vi "ShootRole.vi"(7 "firstCall":bool=TRUE, 8 "error in (no error)":errorcluster, 9 "Robot":refnum<class "Robot.lvclass">, 10 "Game in":refnum<class "Game.lvclass">, 11 "ShootRole in":refnum<class "ShootRole.lvclass">) -> (0 "error out":errorcluster, 1 "Game out":refnum<class "Game.lvclass">, 2 "Robot out":refnum<class "Robot.lvclass">, 3 "ShootRole out":refnum<class "ShootRole.lvclass">)   [LabVIEW 2023, in "ShootRole.lvclass"]
uses:
  ShootRole.lvclass
  Game_class/Game.lvclass
  Robot_class/Robot.lvclass
  Role_class/Role.lvclass/Role.ctl
  ShootTactic_class/States.ctl
  Tacticbook_class/Tacticbook.lvclass/Tacticbook.ctl
  ShootTactic_class/ShootTactic.lvclass/ShootTactic.ctl
  Tacticbook_class/Read ShootTactic.vi
  ShootTactic_class/Read States.vi
  Tacticbook_class/Write ShootTactic.vi
  Role_class/Read Tacticbook.vi
  Role_class/Write Tacticbook.vi
  Role_class/Write tactic_index.vi
  Role_class/Read RobotRef.vi
  Tacticbook_class/Tacticbook.lvclass
  ShootTactic_class/ShootTactic.lvclass
  ShootRole.lvclass/ShootRole.ctl
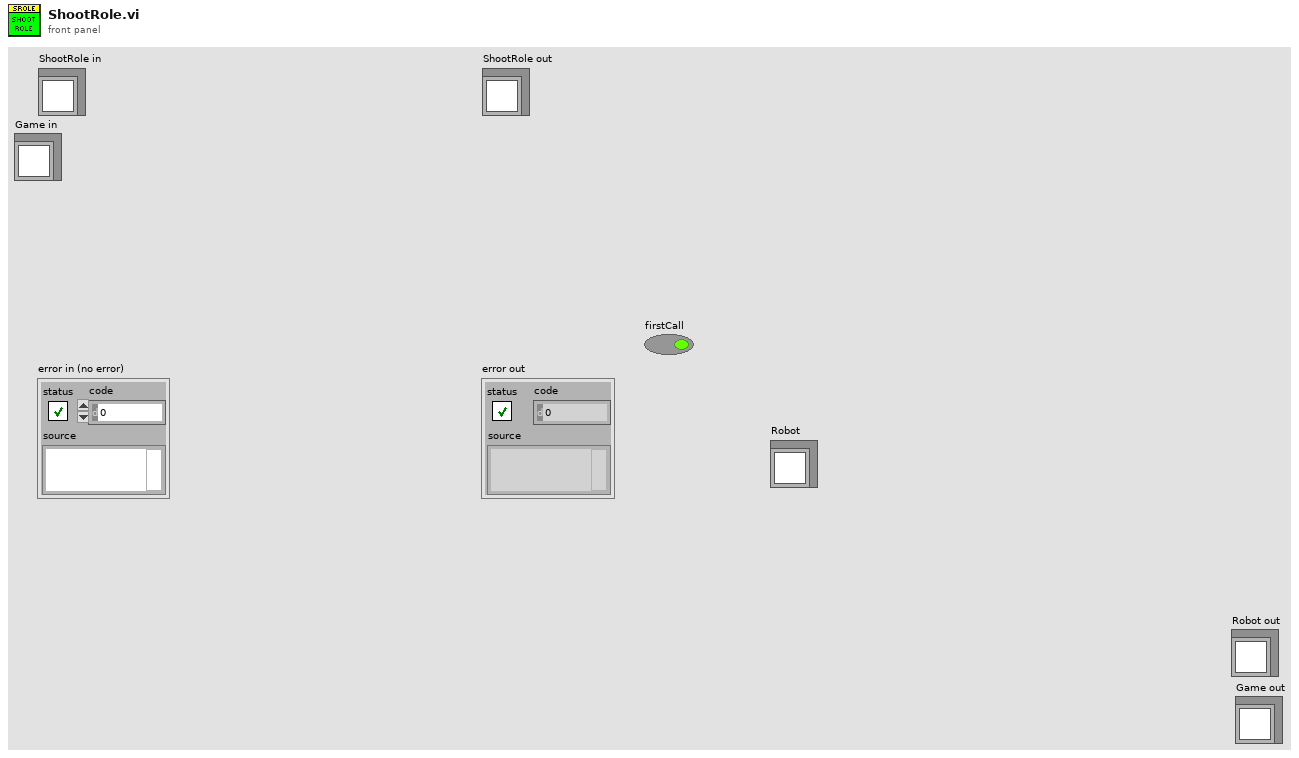
[diagram p1: front panel]
types:
  T1 = typedef "ShootTactic.lvclass/States.ctl" = enum16{"BallInGoalieArea", "Exit", "KickToGoal", "StealBall"}
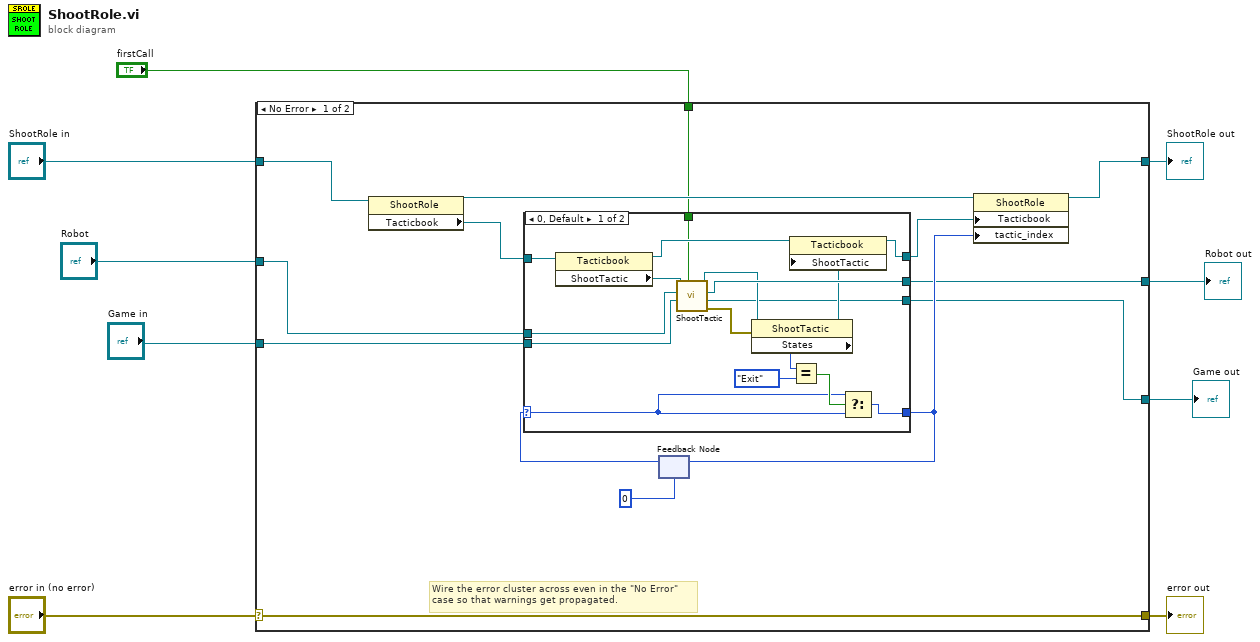
[diagram p0: block diagram]
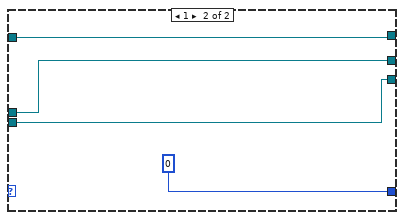
[diagram p2: hidden frame]
diagram:
  n1 = case shown="No Error" "error in (no error)" {
    selector: "error in (no error)" -> [w23 w48]
    tunnel: [w23 w48] -> w8
    tunnel: [w16 w47] -> w7
    tunnel: "ShootRole in" -> [w15 w47]
    tunnel: "Game in" -> [w12 w45]
    tunnel: "Robot" -> [w14 w46]
    tunnel: [w13 w46] -> w4
    tunnel: [w10 w45] -> w3
    tunnel: "firstCall" -> [w11 _]
    frame No Error {
      # "Wire the error cluster across even in the \"No Error\"\ncase so that warnings get propagated."
      n2 = property class="ShootRole"(reference=w15) -> (reference out=w22:refnum<class "ShootRole.lvclass">, "Tacticbook"=w19:refnum<class "Tacticbook.lvclass">)  [unwired: 1 in, 1 out]
      n3 = feedback #1(0) -> (w20:i32)
      n4 = case shown="0, Default" w20 {
        selector: w20 -> [w26 _]
        tunnel: [w32 0] -> w18
        tunnel: w19 -> [w40 w42]
        tunnel: w14 -> [w38 w44]
        tunnel: [w37 w44] -> w13
        tunnel: [w29 w42] -> w17
        tunnel: w12 -> [w28 w41]
        tunnel: w11 -> [w25 _]
        tunnel: [w24 w41] -> w10
        frame 0, Default {
          n5 = property class="Tacticbook"(reference=w40) -> (reference out=w31:refnum<class "Tacticbook.lvclass">, "ShootTactic"=w39:refnum<class "ShootTactic.lvclass">)  [unwired: 1 in, 1 out]
          n6 = call "ShootTactic.vi"("firstCall?"=w25, "Game in"=w28, "Robot"=w38, "ShootTactic in"=w39) -> ("error out"=w36:errorcluster, "Game out"=w24:refnum<class "Game.lvclass">, "Robot out"=w37:refnum<class "Robot.lvclass">, "ShootTactic out"=w35:refnum<class "ShootTactic.lvclass">)  [unwired: 4 in]
          n7 = property class="ShootTactic"(reference=w35, error in=w36) -> (reference out=w30:refnum<class "ShootTactic.lvclass">, "States"=w34:T1)  [unwired: 1 out]
          n8 = property class="Tacticbook"(reference=w31, "ShootTactic"=w30) -> (reference out=w29:refnum<class "Tacticbook.lvclass">)  [unwired: 1 in, 1 out]
          n9 = Equal?(x=w34, y=States."Exit") -> (x = y?=w33:bool)
          n10 = Select(t=w26, s=w33, f=w26) -> (s? t:f=w32:i32)
        }
        frame 1 {
        }
      }
      n11 = feedback-in #1(w18) -> ()
      n12 = property class="ShootRole"(reference=w22, "Tacticbook"=w17, "tactic_index"=w18) -> (reference out=w16:refnum<class "ShootRole.lvclass">)  [unwired: 1 in, 1 out]
    }
    frame Error {
    }
  }
  "error out" <- w8
  "ShootRole out" <- w7
  "Robot out" <- w4
  "Game out" <- w3
